vi "Agilent VNA Convert Form 1 Data.vi"(8 "Raw Data Point":string) -> (0 "Number":cdb)   [LabVIEW 2011]
panel:
  out "Byte Array":i8[](array[numeric])
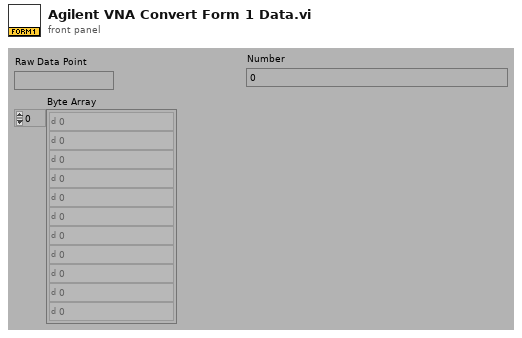
[diagram p1: front panel]
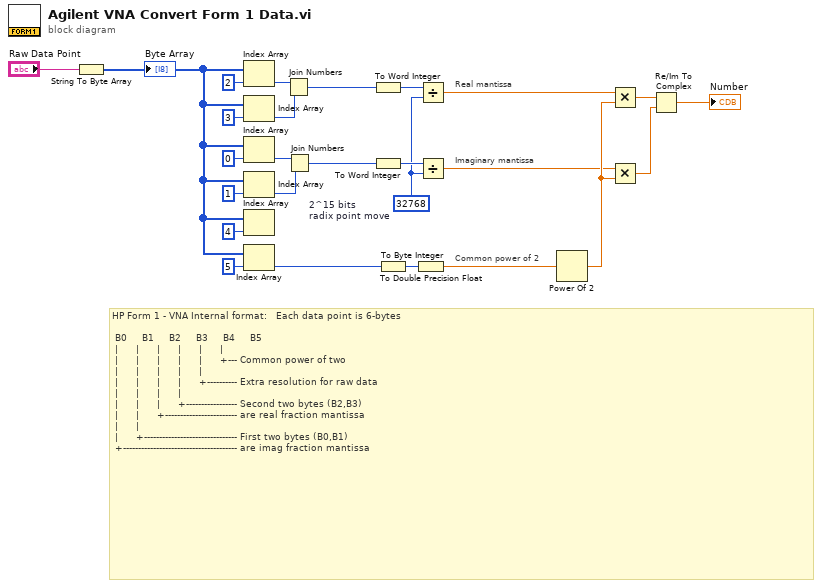
[diagram p0: block diagram]
diagram:
  w10 = u16 32768  # 2^15 bits radix point move
  # "Common power of 2"
  # "Imaginary mantissa"
  # "Real mantissa"
  # "HP Form 1 - VNA Internal format:   Each data point is 6-bytes\n\n B0     B1     B2     B3     B4     B5     \n |      |      |      |      |      |\n |      |      |      |      |      +--- Common power of two\n |      |      |      |      |\n |      |      |      |      +---------- Extra resolution for raw data\n |      |      |      |\n |      |      |      +----------------- Second two bytes (B2,B3)\n |      |      +------------------------ are real fraction mantissa\n |      |\n |      +------------------------------- First two bytes (B0,B1)\n +-------------------------------------- are imag fraction mantissa"
  n1 = String To Byte Array(string="Raw Data Point") -> (unsigned byte array=w7:u8[])
  "Byte Array" <- w7
  n2 = Index Array(array=w7, index=2) -> (element=w5:u8)
  n3 = Index Array(array=w7, index=3) -> (element=w4:u8)
  n4 = Index Array(array=w7, index=0) -> (element=w19:u8)
  n5 = Index Array(array=w7, index=1) -> (element=w18:u8)
  n6 = Index Array(array=w7, index=4) -> ()  [unwired: 1 out]
  n7 = Index Array(array=w7, index=5) -> (element=w14:u8)
  n8 = Join Numbers(hi=w5, lo=w4) -> ((hi.lo)=w6:u16)
  n9 = Join Numbers(hi=w19, lo=w18) -> ((hi.lo)=w17:u16)
  n10 = To Word Integer(number=w6) -> (16bit integer=w12:i16)
  n11 = To Word Integer(number=w17) -> (16bit integer=w11:i16)
  n12 = To Byte Integer(number=w14) -> (8bit integer=w13:i8)
  n13 = To Double Precision Float(number=w13) -> (double precision float=w15:dbl)
  n14 = Divide(x=w12, y=w10) -> (x/y=w8:dbl)
  n15 = Divide(x=w11, y=w10) -> (x/y=w9:dbl)
  n16 = Power Of 2(x=w15) -> (2^x=w16:dbl)
  n17 = Multiply(x=w8, y=w16) -> (x*y=w1:dbl)
  n18 = Multiply(x=w9, y=w16) -> (x*y=w2:dbl)
  n19 = Re/Im To Complex(1:w2, 2:w1) -> (0:→"Number":cdb)
